vi "fix init.vi"(8 "error in":errorcluster, 11 "VI in":refnum<vi>) -> (0 "error out":errorcluster)   [LabVIEW 2013, in "TagBusProcessingPluginFeatureDecider.lvclass"]
uses:
  TagBusProcessingPluginFeatureDecider.lvclass
  <vilib>/Utility/traverseref.llb/TRef TravTarget.ctl
  <vilib>/Utility/traverseref.llb/VI Scripting - Traverse.lvlib
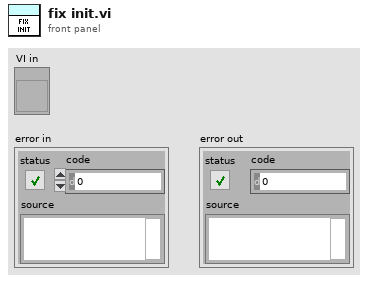
[diagram p1: front panel]
types:
  T1 = typedef "TRef TravTarget.ctl" = enum16{"FP", "BD", "Other"}
  T2 = typedef "ASPM_ArrayOfUniqueIDStringDatanameShortnameLongname.ctl" = T3[]
  T3 = typedef "ASPM_UniqueIDStringDatanameShortnameLongname.ctl" = cluster{"Unique ID string":string, "Data name":string, "Short name (localized)":string, "Long name (localized)":string}
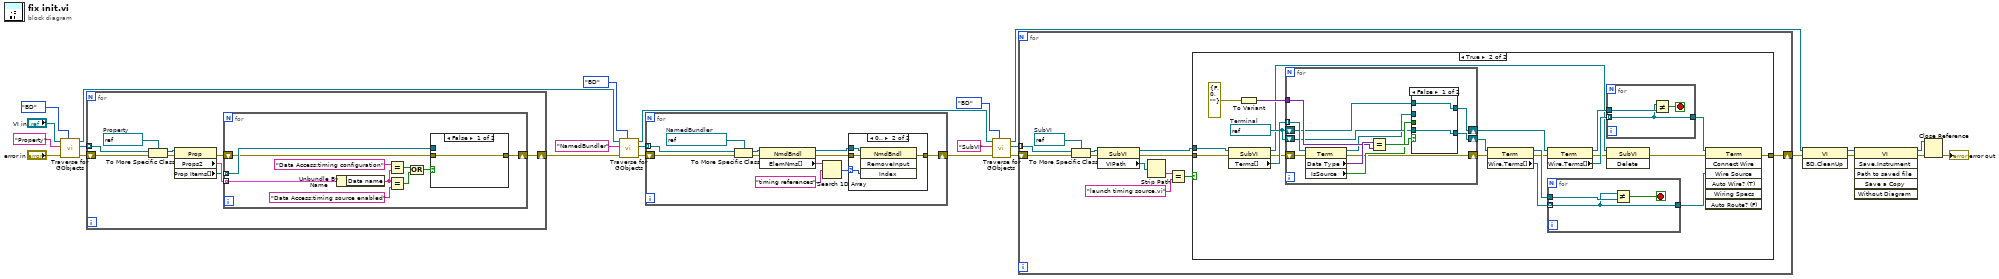
[diagram p0: block diagram]
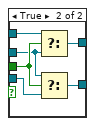
[diagram p3: hidden frame]
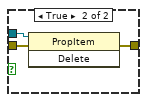
[diagram p4: hidden frame]
diagram:
  n1 = call <vilib>:"Traverse for GObjects.vi"("Traverse Target"=TRef_TravTarget."BD", "error in (no error)"="error in", "Class Name"="Property", "VI Refnum"="VI in") -> ("error out"=w13:errorcluster, "References"=w12:refnum<vi>[], "dup VI Refnum"=w10:refnum<vi>)  [unwired: 4 in, 1 out]
  n2 = for {
    shift-right: [w28] -> w11
    shift-left: w13 -> [w32]
    tunnel: w12 -> [w34] mode=indexing
    w33 = refnum<vi> refnum  # Property
    n3 = To More Specific Class(target class=w33, reference=w34, error in=w32) -> (specific class reference=w31:refnum<vi>, error out=w30:errorcluster)
    n4 = property class="Prop"(reference=w31, error in=w30) -> (error out=w29:errorcluster, "Props2"=w27:T2, "Prop Items[]"=w26:refnum<vi>[])  [unwired: 1 out]
    n5 = for {
      shift-right: [w41] -> w28
      shift-left: w29 -> [w40]
      tunnel: w27 -> [w44] mode=indexing
      tunnel: w26 -> [w42] mode=indexing
      n6 = Unbundle By Name(w44) -> ("Data name"=w39:string)
      n7 = Equal?(x="Data Access:timing configuration", y=w39) -> (x = y?=w36:bool)
      n8 = Equal?(x=w39, y="Data Access:timing source enabled" ("x")) -> (x = y?=w37:bool)
      n9 = Or(x=w36, y=w37) -> (x .or. y?=w35:bool)
      n10 = case shown="False" w35 {
        tunnel: w42 -> [_ w48]
        tunnel: [w45 w47] -> w41
        tunnel: w40 -> [w45 w46]
        frame False {
        }
        frame True {
          n11 = invoke class="PropItem" method="Delete"(reference=w48, error in=w46) -> (error out=w47:errorcluster)  [unwired: 1 in, 2 out]
        }
      }
    }
  }
  n12 = call <vilib>:"Traverse for GObjects.vi"("Traverse Target"=TRef_TravTarget."BD", "error in (no error)"=w11, "Class Name"="NamedBundler", "VI Refnum"=w10) -> ("error out"=w9:errorcluster, "References"=w17:refnum<vi>[], "dup VI Refnum"=w3:refnum<vi>)  [unwired: 4 in, 1 out]
  n13 = for {
    tunnel: w17 -> [w58] mode=indexing
    shift-right: [w50] -> w4
    shift-left: w9 -> [w55]
    w59 = refnum<vi> refnum  # NamedBundler
    n14 = To More Specific Class(target class=w59, reference=w58, error in=w55) -> (specific class reference=w57:refnum<vi>, error out=w56:errorcluster)
    n15 = property class="NmdBndl"(reference=w57, error in=w56) -> (reference out=w54:refnum<vi>, error out=w51:errorcluster, "ElemNms[]"=w53:string[])
    n16 = Search 1D Array(1D array=w53, element="timing references") -> (index of element=w49:i32)  [unwired: 1 in]
    n17 = case shown="0.." w49 {
      selector: w49 -> [_ w61]
      tunnel: w54 -> [_ w64]
      tunnel: w51 -> [w60 w63]
      tunnel: [w60 w62] -> w50
      frame ..-1 {
      }
      frame 0.. {
        n18 = invoke class="NmdBndl" method="RemoveInput"(reference=w64, error in=w63, "Index"=w61) -> (error out=w62:errorcluster)  [unwired: 1 in, 3 out]
      }
    }
  }
  n19 = call <vilib>:"Traverse for GObjects.vi"("Traverse Target"=TRef_TravTarget."BD", "error in (no error)"=w4, "Class Name"="SubVI", "VI Refnum"=w3) -> ("error out"=w8:errorcluster, "References"=w6:refnum<vi>[], "dup VI Refnum"=w2:refnum<vi>)  [unwired: 4 in, 1 out]
  n20 = for {
    tunnel: w6 -> [w75] mode=indexing
    shift-right: [w69] -> w1
    shift-left: w8 -> [w72]
    w76 = refnum<vi> refnum  # SubVI
    n21 = To More Specific Class(target class=w76, reference=w75, error in=w72) -> (specific class reference=w74:refnum<vi>, error out=w73:errorcluster)
    n22 = property class="SubVI"(reference=w74, error in=w73) -> (reference out=w71:refnum<vi>, error out=w70:errorcluster, "VIPath"=w68:path)
    n23 = Strip Path(path=w68) -> (name=w67:string)  [unwired: 1 out]
    n24 = Equal?(x=w67, y="launch timing source.vi") -> (x = y?=w65:bool)
    n25 = case shown="True" w65 {
      tunnel: w71 -> [_ w98]
      tunnel: w70 -> [w77 w97]
      tunnel: [w77 w78] -> w69
      frame False {
      }
      frame True {
        w92 = refnum<vi> refnum  # Terminal
        n26 = property class="SubVI"(reference=w98, error in=w97) -> (reference out=w81:refnum<vi>, error out=w93:errorcluster, "Terms[]"=w96:refnum<vi>[])
        n27 = To Variant(anything=errorcluster {"status"=FALSE, "code"=0, "source"=""} ("error constant")) -> (Variant=w94:variant)
        n28 = for {
          tunnel: w96 -> [w116] mode=indexing
          tunnel: w94 -> [w114]
          shift-right: [w106] -> w91
          shift-left: w93 -> [w113]
          shift-right: [w110] -> w90
          shift-left: w92 -> [w109]
          shift-right: [w108] -> w85
          shift-left: w92 -> [w107]
          n29 = property class="Term"(reference=w116, error in=w113) -> (reference out=w105:refnum<vi>, error out=w106:errorcluster, "Data Type"=w115:variant, "IsSource"=w111:bool)
          n30 = Equal?(x=w115, y=w114) -> (x = y?=w112:bool)
          n31 = case shown="False" w112 {
            tunnel: w111 -> [_ w122]
            tunnel: [w118 w123] -> w110
            tunnel: w109 -> [w118 w124]
            tunnel: [w117 w119] -> w108
            tunnel: w107 -> [w117 w120]
            tunnel: w105 -> [_ w121]
            frame False {
            }
            frame True {
              n32 = Select(t=w120, s=w122, f=w121) -> (s? t:f=w119:refnum<vi>)
              n33 = Select(t=w121, s=w122, f=w124) -> (s? t:f=w123:refnum<vi>)
            }
          }
        }
        n34 = property class="Term"(reference=w90, error in=w91) -> (reference out=w88:refnum<vi>, error out=w84:errorcluster, "Wire.Terms[]"=w89:refnum<vi>[])
        n35 = property class="Term"(reference=w85, error in=w84) -> (reference out=w87:refnum<vi>, error out=w80:errorcluster, "Wire.Terms[]"=w86:refnum<vi>[])
        n36 = for {
          tunnel: w89 -> [w102] mode=indexing
          tunnel: w88 -> [w104]
          tunnel: [w102] -> w79
          stop <- w103 stop-if-true
          n37 = Not Equal?(x=w102, y=w104) -> (x != y?=w103:bool)
        }
        n38 = for {
          tunnel: w86 -> [w99] mode=indexing
          tunnel: w87 -> [w101]
          tunnel: [w99] -> w83
          stop <- w100 stop-if-true
          n39 = Not Equal?(x=w99, y=w101) -> (x != y?=w100:bool)
        }
        n40 = invoke class="SubVI" method="Delete"(reference=w81, error in=w80) -> (error out=w82:errorcluster)  [unwired: 1 in, 2 out]
        n41 = invoke class="Term" method="Connect Wire"(reference=w83, error in=w82, "Wire Source"=w79) -> (error out=w78:errorcluster)  [unwired: 4 in, 6 out]
      }
    }
  }
  n42 = invoke class="VI" method="BD.CleanUp"(reference=w2, error in=w1) -> (reference out=w14:refnum<vi>, error out=w15:errorcluster)  [unwired: 1 in, 1 out]
  n43 = invoke class="VI" method="Save.Instrument"(reference=w14, error in=w15) -> (reference out=w21:refnum<vi>, error out=w23:errorcluster)  [unwired: 4 in, 4 out]
  n44 = Close Reference(reference=w21, error in (no error)=w23) -> (error out=→"error out":errorcluster)
